vi "Header Footer Modify Image Cell.vi"(2 "Header or Footer":T1, 5 "Modify Image Cell":bool, 9 "Header or Footer Complete Cluster IN":T2, 11 "error in (no error)":errorcluster) -> (10 "Header or Footer Complete Cluster OUT":T2, 15 "error out":errorcluster)   [LabVIEW 2019]
doc: "Version 1.0\nDeveloped by Jean-Marc Simard\nCopyright © 2010, Exaprom Inc.\nAll rights reserved.\nLicense: BSD\n\nWith iTextSharp 4.1.6 (http://itextsharp.sourceforge.net)\nunder Mozilla Public License Version 1.1\n(http://www.mozilla.org/MPL/MPL-1.1.html)"
uses:
  <userlib>/Exaprom PDF/Controls/Header, Footer and Watermark Controls/Header Footer Complete Cluster.ctl
  <userlib>/Exaprom PDF/Controls/Header, Footer and Watermark Controls/Header or Footer Position.ctl
  <userlib>/Exaprom PDF/Controls/Header, Footer and Watermark Controls/Header Footer Cluster with references.ctl
  <userlib>/Exaprom PDF/Controls/Header, Footer and Watermark Controls/Header Footer Type.ctl
  <userlib>/Exaprom PDF/Controls/Header, Footer and Watermark Controls/Header footer horiz alignment.ctl
  <userlib>/Exaprom PDF/Controls/Table Controls/Cell Vertical alignment.ctl
  <userlib>/Exaprom PDF/Controls/Header, Footer and Watermark Controls/Page number.ctl
  C:/Program Files/National Instruments/LabVIEW 2019/user.lib/Exaprom PDF/DLL/itextsharp.dll
  DLL/itextsharp.dll
  <userlib>/Exaprom PDF/Controls/Font Controls/Font complete cluster horizontal.ctl
  <userlib>/Exaprom PDF/Controls/Font Controls/Font size.ctl
  <userlib>/Exaprom PDF/Controls/Font Controls/Font color.ctl
  <userlib>/Exaprom PDF/Controls/Font Controls/Type and encoding.ctl
  <userlib>/Exaprom PDF/Controls/Text Controls/Unicode/Type and run direction.ctl
  <userlib>/Exaprom PDF/Controls/Header, Footer and Watermark Controls/Header Footer Line.ctl
  <userlib>/Exaprom PDF/Controls/Text Controls/Line spacing.ctl
  <userlib>/Exaprom PDF/Controls/Header, Footer and Watermark Controls/Header or Footer.ctl
  <userlib>/Exaprom PDF/Controls/Image Controls/Image Scale Type.ctl
panel:
  # "X"
  # "Y"
  # "X"
  # "Y"
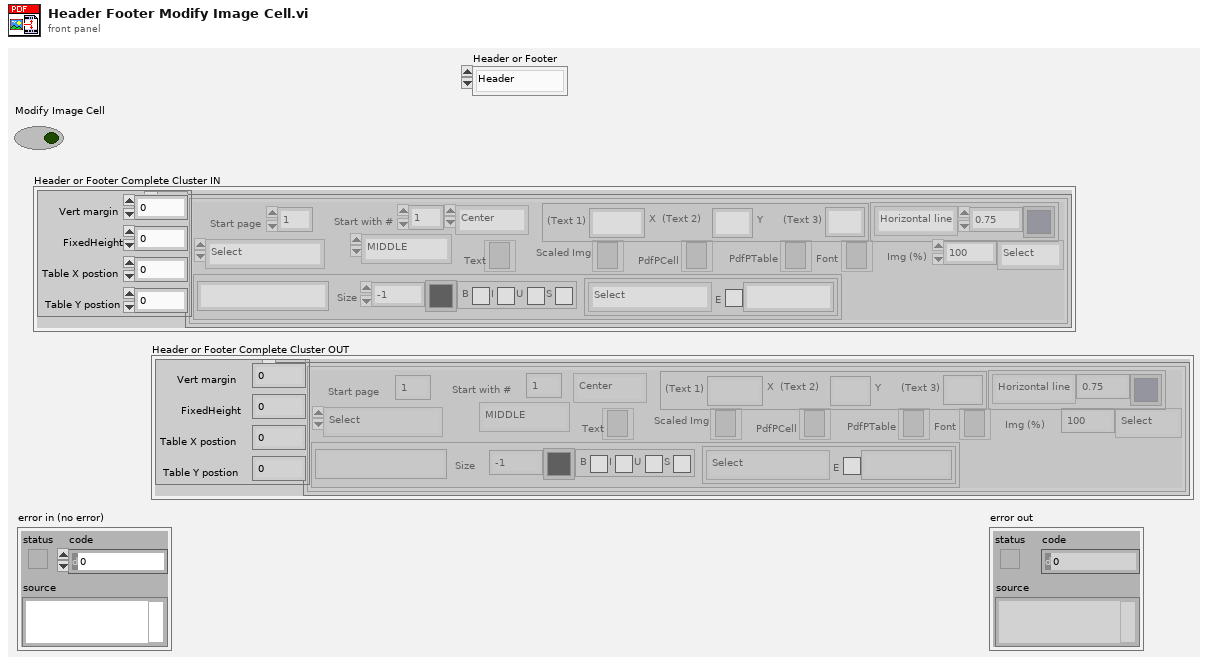
[diagram p1: front panel]
types:
  T1 = typedef "Header or Footer.ctl" = enum16{"Header", "Footer"}
  T2 = typedef "Header Footer Complete Cluster.ctl" = cluster{"Table position":T3, "Header Footer Cluster with references [ ]":T4[]}
  T3 = typedef "Header or Footer Position.ctl" = cluster{"Vert margin":dbl, "FixedHeight":dbl, "Table X postion":dbl, "Table Y postion":dbl}
  T4 = typedef "Header Footer Cluster with references.ctl" = cluster{"Start page":i32, "Type":T5, "Start with #":i32, "Alignment":T6, "Vertical Alignement":T7, "Page #":T8, "Text":refnum<k24>, "Scaled Img":refnum<k24>, "PdfPCell":refnum<k24>, "PdfPTable":refnum<k24>, "Font Cluster":T9, "Font ":refnum<k24>, "Img (%)":sgl, "Line":cluster{"Line":T14, "Thickness (points)":sgl, "Colour":T11}, "Line spacing":T15}
  T5 = typedef "Header Footer Type.ctl" = enum16{"Select", "Text", "Text + hyperlink", "Page number", "Image", "Image + hyperlink"}
  T6 = typedef "Header footer horiz alignment.ctl" = enum16{"Left", "Center", "Right"}
  T7 = typedef "Cell Vertical alignment.ctl" = enum16{"TOP", "MIDDLE", "BOTTOM"}
  T8 = typedef "Page number.ctl" = cluster{"Text 1":string, "Text 2":string, "Text 3":string}
  T9 = typedef "Font complete cluster horizontal.ctl" = cluster{"Name":string, "Size":T10, "Color":T11, "Style":cluster{"Bold":bool, "Italic":bool, "Underline":bool, "Strikeout":bool}, "Type":T12}
  T10 = typedef "Font size.ctl" = sgl
  T11 = typedef "Font color.ctl" = u32
  T12 = typedef "Type and encoding.ctl" = cluster{"Type&direction":T13, "Embedded":bool, "Encoding":string}
  T13 = typedef "Type and run direction.ctl" = enum16{"Select", "ASCII", "UTF-16", "UTF-16 (default)", "UTF-16 (LTR)", "UTF-16 (RTL)"}
  T14 = typedef "Header Footer Line.ctl" = enum16{"No line", "Horizontal line"}
  T15 = typedef "Line spacing.ctl" = enum16{"Select", "1.0", "1.5", "2.0"}
  T16 = typedef "Image Scale Type.ctl" = enum16{"%", "Height", "Width"}
  T17 = cluster{"Table position":T3, "Header Footer Cluster with references [ ]":T4[]}
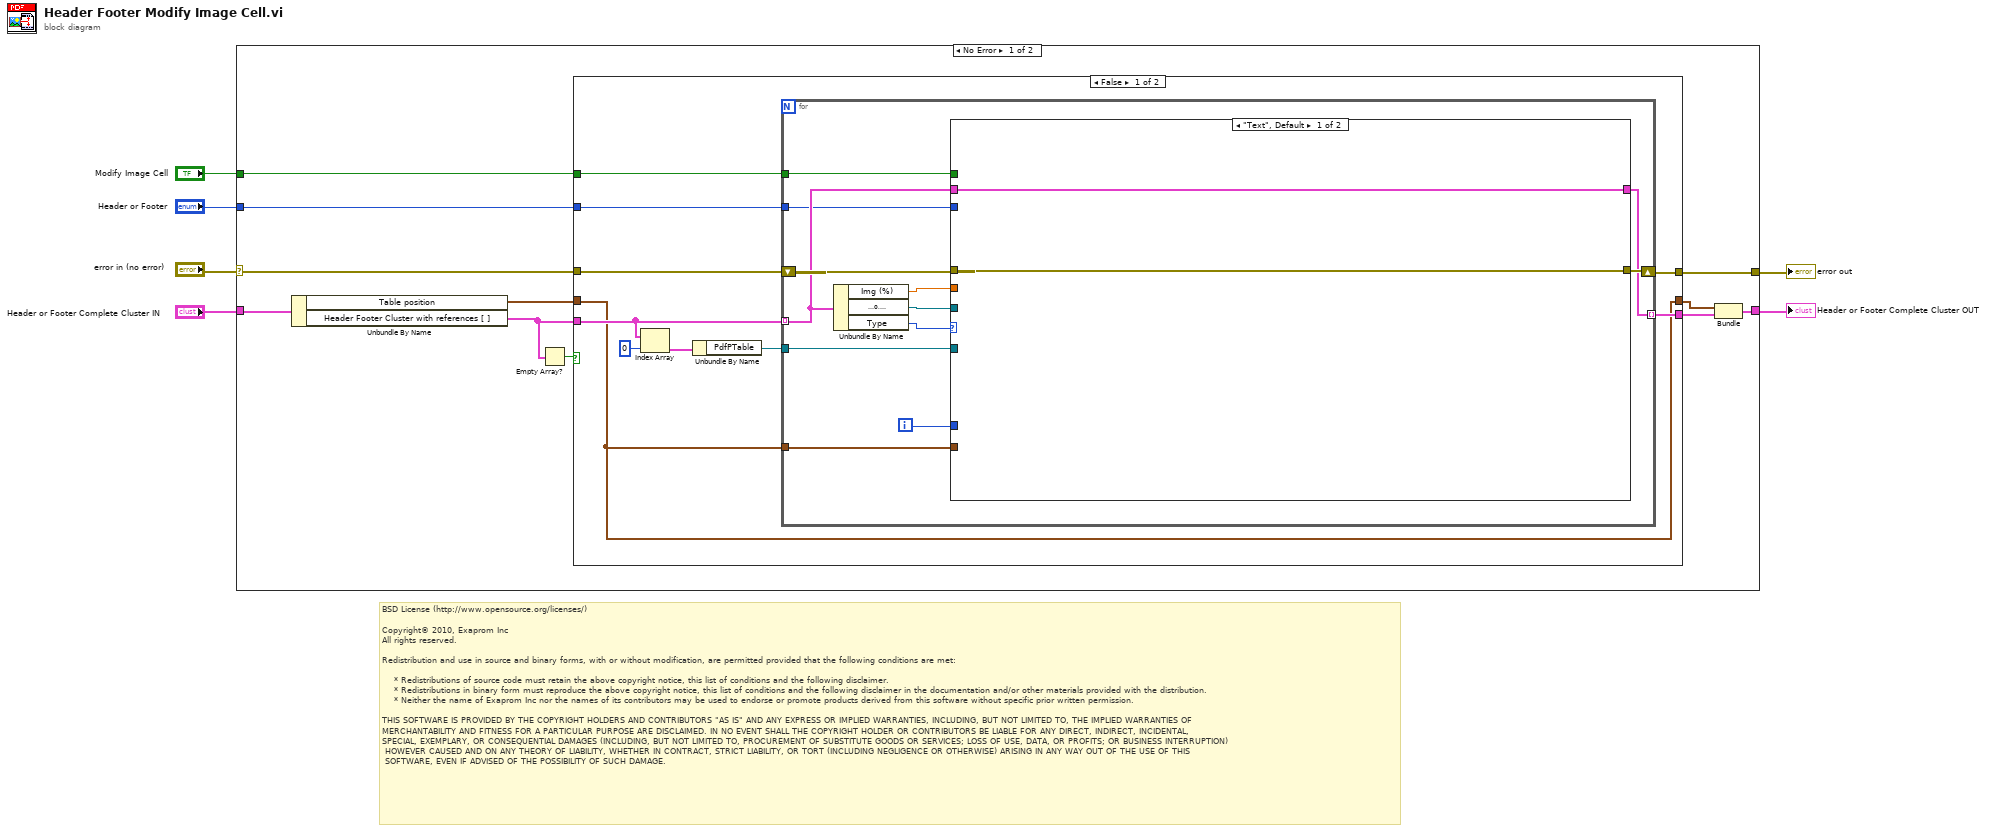
[diagram p0: block diagram]
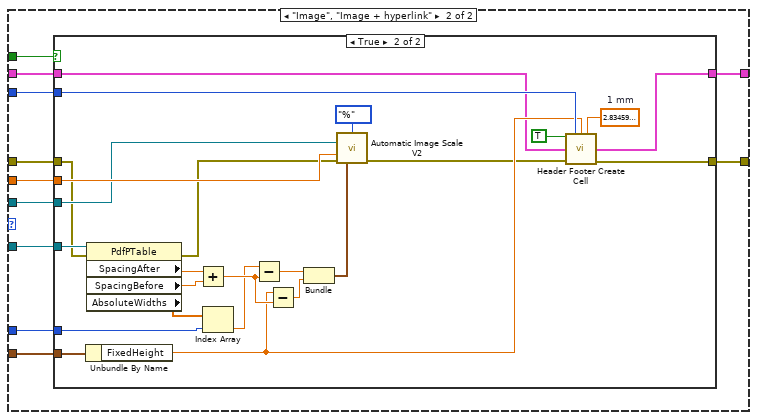
[diagram p2: hidden frame]
diagram:
  # "BSD License (http://www.opensource.org/licenses/)\n\nCopyright© 2010, Exaprom Inc\nAll rights reserved.\n\nRedistribution and use in source and binary forms, with or without modification, are permitted provided that the following conditions are met:\n\n    * Redistributions of source code must retain the above copyright notice, this list of conditions and the following disclaimer.\n    * Redistributions in binary form must reproduce the above copyright notice, this list of conditions and the following disclaimer in the documentation and/or other materials provided with the distribution.\n    * Neither the name of Exaprom Inc nor the names of its contributors may be used to endorse or promote products derived from this software without specific prior written permission.\n\nTHIS SOFTWARE IS PROVIDED BY THE COPYRIGHT HOLDERS AND CONTRIBUTORS \"AS IS\" AND ANY EXPRESS OR IMPLIED WARRANTIES, INCLUDING, BUT NOT LIMITED TO, THE IMPLIED WARRANTIES OF \nMERCHANTABILITY AND FITNESS FOR A PARTICULAR PURPOSE ARE DISCLAIMED. IN NO EVENT SHALL THE COPYRIGHT HOLDER OR CONTRIBUTORS BE LIABLE FOR ANY DIRECT, INDIRECT, INCIDENTAL,\nSPECIAL, EXEMPLARY, OR CONSEQUENTIAL DAMAGES (INCLUDING, BUT NOT LIMITED TO, PROCUREMENT OF SUBSTITUTE GOODS OR SERVICES; LOSS OF USE, DATA, OR PROFITS; OR BUSINESS INTERRUPTION)\n HOWEVER CAUSED AND ON ANY THEORY OF LIABILITY, WHETHER IN CONTRACT, STRICT LIABILITY, OR TORT (INCLUDING NEGLIGENCE OR OTHERWISE) ARISING IN ANY WAY OUT OF THE USE OF THIS\n SOFTWARE, EVEN IF ADVISED OF THE POSSIBILITY OF SUCH DAMAGE."
  n1 = case shown="No Error" "error in (no error)" {
    selector: "error in (no error)" -> [w16 w83]
    tunnel: "Header or Footer Complete Cluster IN" -> [w15 w82]
    tunnel: [w17 w83] -> w6
    tunnel: [w14 w82] -> w2
    tunnel: "Header or Footer" -> [w13 _]
    tunnel: "Modify Image Cell" -> [w10 _]
    frame No Error {
      n2 = Unbundle By Name(w15) -> ("Table position"=w11:T3, "Header Footer Cluster with references [ ]"=w7:T4[])
      n3 = Empty Array?(array=w7) -> (empty?=w8:bool)
      n4 = case shown="False" w8 {
        tunnel: [w27 w81] -> w17
        tunnel: w16 -> [w26 w81]
        tunnel: w7 -> [w22 w80]
        tunnel: w13 -> [w21 _]
        tunnel: [w20 w80] -> w12
        tunnel: w11 -> [w18 w79]
        tunnel: w10 -> [w19 _]
        tunnel: [w18 w79] -> w9
        frame False {
          n5 = Index Array(array=w22, index=0) -> (element=w24:T4)
          n6 = Unbundle By Name(w24) -> ("PdfPTable"=w23:refnum<k24>)
          n7 = for {
            tunnel: w22 -> [w32] mode=indexing
            tunnel: w23 -> [w35]
            tunnel: w18 -> [w37]
            shift-right: [w30] -> w27
            shift-left: w26 -> [w38]
            tunnel: w21 -> [w31]
            tunnel: [w29] -> w20 mode=indexing
            tunnel: w19 -> [w28]
            i -> [w36]
            n8 = Unbundle By Name(w32) -> ("Img (%)"=w33:sgl, "Scaled Img"=w34:refnum<k24>, "Type"=w39:T5)
            n9 = case shown="\"Text\", Default" w39 {
              tunnel: w38 -> [w40 w52]
              tunnel: [w40 w51] -> w30
              tunnel: w35 -> [_ w50]
              tunnel: w36 -> [_ w49]
              tunnel: w37 -> [_ w48]
              tunnel: w34 -> [_ w47]
              tunnel: w33 -> [_ w46]
              tunnel: w32 -> [w41 w45]
              tunnel: w31 -> [_ w44]
              tunnel: [w41 w43] -> w29
              tunnel: w28 -> [_ w42]
              frame "Text", Default {
              }
              frame "Image", "Image + hyperlink" {
                n10 = case shown="True" w42 {
                  tunnel: w46 -> [_ w78]
                  tunnel: w52 -> [w54 w65]
                  tunnel: [w54 w63] -> w51
                  tunnel: w50 -> [_ w77]
                  tunnel: w49 -> [_ w76]
                  tunnel: w48 -> [_ w68]
                  tunnel: w47 -> [_ w66]
                  tunnel: w45 -> [w53 w58]
                  tunnel: w44 -> [_ w61]
                  tunnel: [w53 w57] -> w43
                  frame False {
                  }
                  frame True {
                    w62 = sgl 2.8346  # 1 mm
                    n11 = Unbundle By Name(w68) -> ("FixedHeight"=w60:dbl)
                    n12 = property class="PdfPTable"(reference=w77, error in=w65) -> (error out=w64:errorcluster, "SpacingAfter"=w72:sgl, "SpacingBefore"=w71:sgl, "AbsoluteWidths"=w75:sgl[])  [unwired: 1 out]
                    n13 = Add(x=w72, y=w71) -> (x+y=w70:sgl)
                    n14 = Index Array(array=w75, index=w76) -> (element=w69:sgl)
                    n15 = Subtract(x=w69, y=w70) -> (x-y=w74:sgl)
                    n16 = Subtract(x=w60, y=w70) -> (x-y=w73:dbl)
                    n17 = Bundle(w74, w73) -> (w67:cluster{sgl, dbl})  [unwired: 1 out]
                    n18 = call <userlib>:"Automatic Image Scale V2.vi"("Scale Type"=Image_Scale_Type."%", "GetInstanceImage IN"=w66, "Scale percent IN"=w78, "error in (no error)"=w64, "Box"=w67) -> ("error out"=w55:errorcluster)  [unwired: 6 in, 4 out]
                    n19 = call <userlib>:"Header Footer Create Cell.vi"("Change format?"=TRUE, "Header or Footer"=w61, "FixedHeight (points)"=w60, "Padding (points)"=w62, "Header Footer Cluster with references IN"=w58, "error in (no error)"=w55) -> ("Header Footer Cluster with references OUT"=w57:T4, "error out"=w63:errorcluster)  [unwired: 2 in, 6 out]
                  }
                }
              }
            }
          }
        }
        frame True {
        }
      }
      n20 = Bundle("Table position"=w9, "Header Footer Cluster with references [ ]"=w12) -> (w14:T17)  [unwired: 1 out]
    }
    frame Error {
    }
  }
  "error out" <- w6
  "Header or Footer Complete Cluster OUT" <- w2
